vi "Newton's method.vi"(1 "Max Iterations (1,000)":i32=1000, 2 "Initial Guess":dbl, 4 "Function Reference":refnum<vi>) -> (0 "x_n":dbl)   [LabVIEW 2020, in "Automatic Differentiation.lvlib"]
uses:
  libraries/Automatic Differentiation/Automatic Differentiation.lvlib
  Dual.lvclass
  Dual.lvclass/Dual.ctl
  Dual to Double.vi
  libraries/Automatic Differentiation/Evaluate Function.vi/9b1629ae-3de0-49eb-9b0a-cc9e581fb6c0.vi
  Add infinitesimal to Double.vi
  Read Dual Part.vi
  libraries/Automatic Differentiation/Evaluate Function.vi/9b1629ae-3de0-49eb-9b0a-cc9e581fb6c0.vi/5957e011-cf56-4527-b6ed-13c3a4ca997b.vi
  Write a.vi
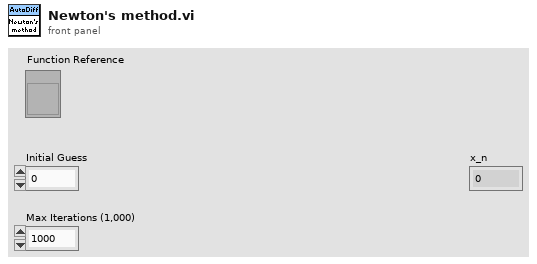
[diagram p1: front panel]
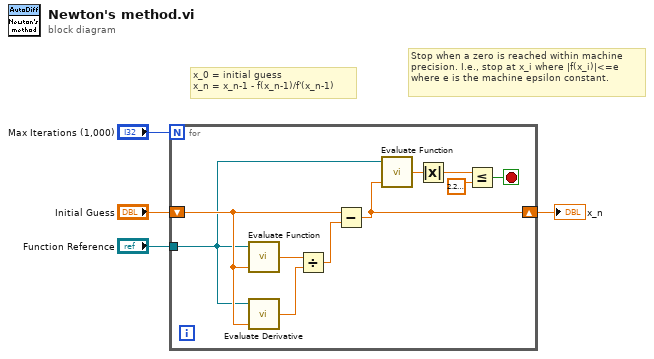
[diagram p0: block diagram]
diagram:
  # "Stop when a zero is reached within machine precision. I.e., stop at x_i where |f(x_i)|<=e where e is the machine epsilon constant."
  # "x_0 = initial guess\nx_n = x_n-1 - f(x_n-1)/f'(x_n-1)"
  n1 = for {
    N: "Max Iterations (1,000)" -> [_]
    tunnel: "Function Reference" -> [w10]
    shift-right: [w9] -> w2
    shift-left: "Initial Guess" -> [w11]
    stop <- w5 stop-if-true
    n2 = call "Evaluate Function.vi"("x"=w11, "Function Reference"=w10) -> ("f(x)"=w14:dbl)  [unwired: 1 in]
    n3 = call "Evaluate Derivative.vi"("x"=w11, "Function Reference"=w10) -> ("f'(x)"=w13:dbl)  [unwired: 1 in]
    n4 = Divide(x=w14, y=w13) -> (x/y=w12:dbl)
    n5 = Subtract(x=w11, y=w12) -> (x-y=w9:dbl)
    n6 = call "Evaluate Function.vi"("x"=w9, "Function Reference"=w10) -> ("f(x)"=w8:dbl)  [unwired: 1 in]
    n7 = Absolute Value(x=w8) -> (abs(x)=w7:dbl)
    n8 = Less Or Equal?(x=w7, y=2.220446049250313e-16) -> (x <= y?=w5:bool)
  }
  "x_n" <- w2
